vi "PentaPanesDemo.vi"() -> ()   [LabVIEW 2022 SP3]
uses:
  PentaPanesClassLibrary.lvlibp/PanesColors.ctl
  <vilib>/Utility/miscctls.llb/LVBoundsTypeDef.ctl
  Tools/Type Defs/XYZ Indicators.ctl
  Tools/Type Defs/XYZ Controls.ctl
  Tools/Type Defs/XYZ ControlButtonsMini.ctl
  PentaPanesClassLibrary.lvlibp/ResizeBehaviourCluster.ctl
  PentaPanesClassLibrary.lvlibp/BordersCluster.ctl
  PentaPanesClassLibrary.lvlibp/PanePosition.ctl
  <vilib>/Platform/browser.llb/Open URL in Default Browser (string).vi
  PentaPanesClassLibrary.lvlibp/PentaPanes.lvclass
  PentaPanesClassLibrary.lvlibp/1abvi3w/vi.lib/Utility/miscctls.llb/LVBoundsTypeDef.ctl
  PentaPanesClassLibrary.lvlibp
panel:
  out "Logo":picture[](array[picture])
  out "Icons Values":bool[](array[boolean])
  out "IconNames":string[](array[string])
  out "Icons":picture[](array[picture])=[bytes[7230], bytes[7230], bytes[7230], bytes[7230], bytes[7230], bytes[7230], bytes[7230], bytes[7230], bytes[7230], bytes[7230], bytes[7230], bytes[7230], bytes[7230], bytes[7230], bytes[7230], bytes[7230], bytes[7230], bytes[7230], bytes[7230], bytes[7230], bytes[7230], bytes[7230], bytes[7230], bytes[7230], bytes[7230], bytes[7230], bytes[7230], bytes[7230], bytes[7230], bytes[7230], bytes[7230], bytes[7230], bytes[7230], bytes[7230], bytes[7230], bytes[7230], bytes[7230], bytes[7230], bytes[7230], bytes[7230], bytes[7230], bytes[7230], bytes[7230], bytes[7230], bytes[7230], bytes[7230], bytes[7230], bytes[7230], bytes[7230], bytes[7230], bytes[7230], bytes[7230]]
  in  "Options Tree":string[](tree)=["About"]
  in  "Options Tab":T1(tab)
  in  "Developed By\nLEAP CODE\nLinking hardware \nwith software\n\nYoni Cohen":string="yoncoh@gmail.com"
  in  "Icon set by":string="https://icons8.com"
  out "about picture":picture
  in  "Graphs Layout":T2(ring)=enum."3 Line graphs"
  in  "Right Pane View":u16(ring) items=["Simple GUI SubVI", "Positioner", "Debug"]
  in  "Top Pane Size":i32=75 caption="Top"
  in  "Right Pane Size":i32=156 caption="Right" max=4000
  in  "Left Pane Size":i32=113 caption="Left"
  in  "Bottom Pane Size":i32=100 caption="Bottom"
  in  "Colors":T3
  out "Intensity Graph 2":dbl[][](graph)
  out "XY Graph 3":cluster{dbl[], dbl[]}[](graph)
  out "XY Graph 2":cluster{dbl[], dbl[]}[](graph)
  out "XY Graph":cluster{dbl[], dbl[]}[](graph)
  out "Intensity Graph":dbl[][](graph)
  in  "Debug Tab":enum32{"Page 1", "Page 2"}(tab)
  out "Init Error":errorcluster
  out "Eventloop Error":errorcluster
  out "App Path":path=path "E:/Work/5PanesWindow/5PanesDemo.vi"
  out "FP Bounds":T4
  in  "Positioner":enum32{"Page 1", "Page 2"}(tab)
  in  "Directions Cluster 2":T5
  in  "GO Button":bool
  in  "POS 2":T6
  out "POS":T7
  in  "Listbox":i32(listbox)=-1
  # "Overview: A mockup of a GUI window demonstrating the use of \nthe \"PentaPanes\" Class\nRequirements: LabVIEW 2023 or \ncompatible \nInstructions: Run this VI and play \naround with the GUI. \nopen and close panes by pressing the white splitters."
  # "Panes"
  # "Sizes"
  # "Debug Pane"
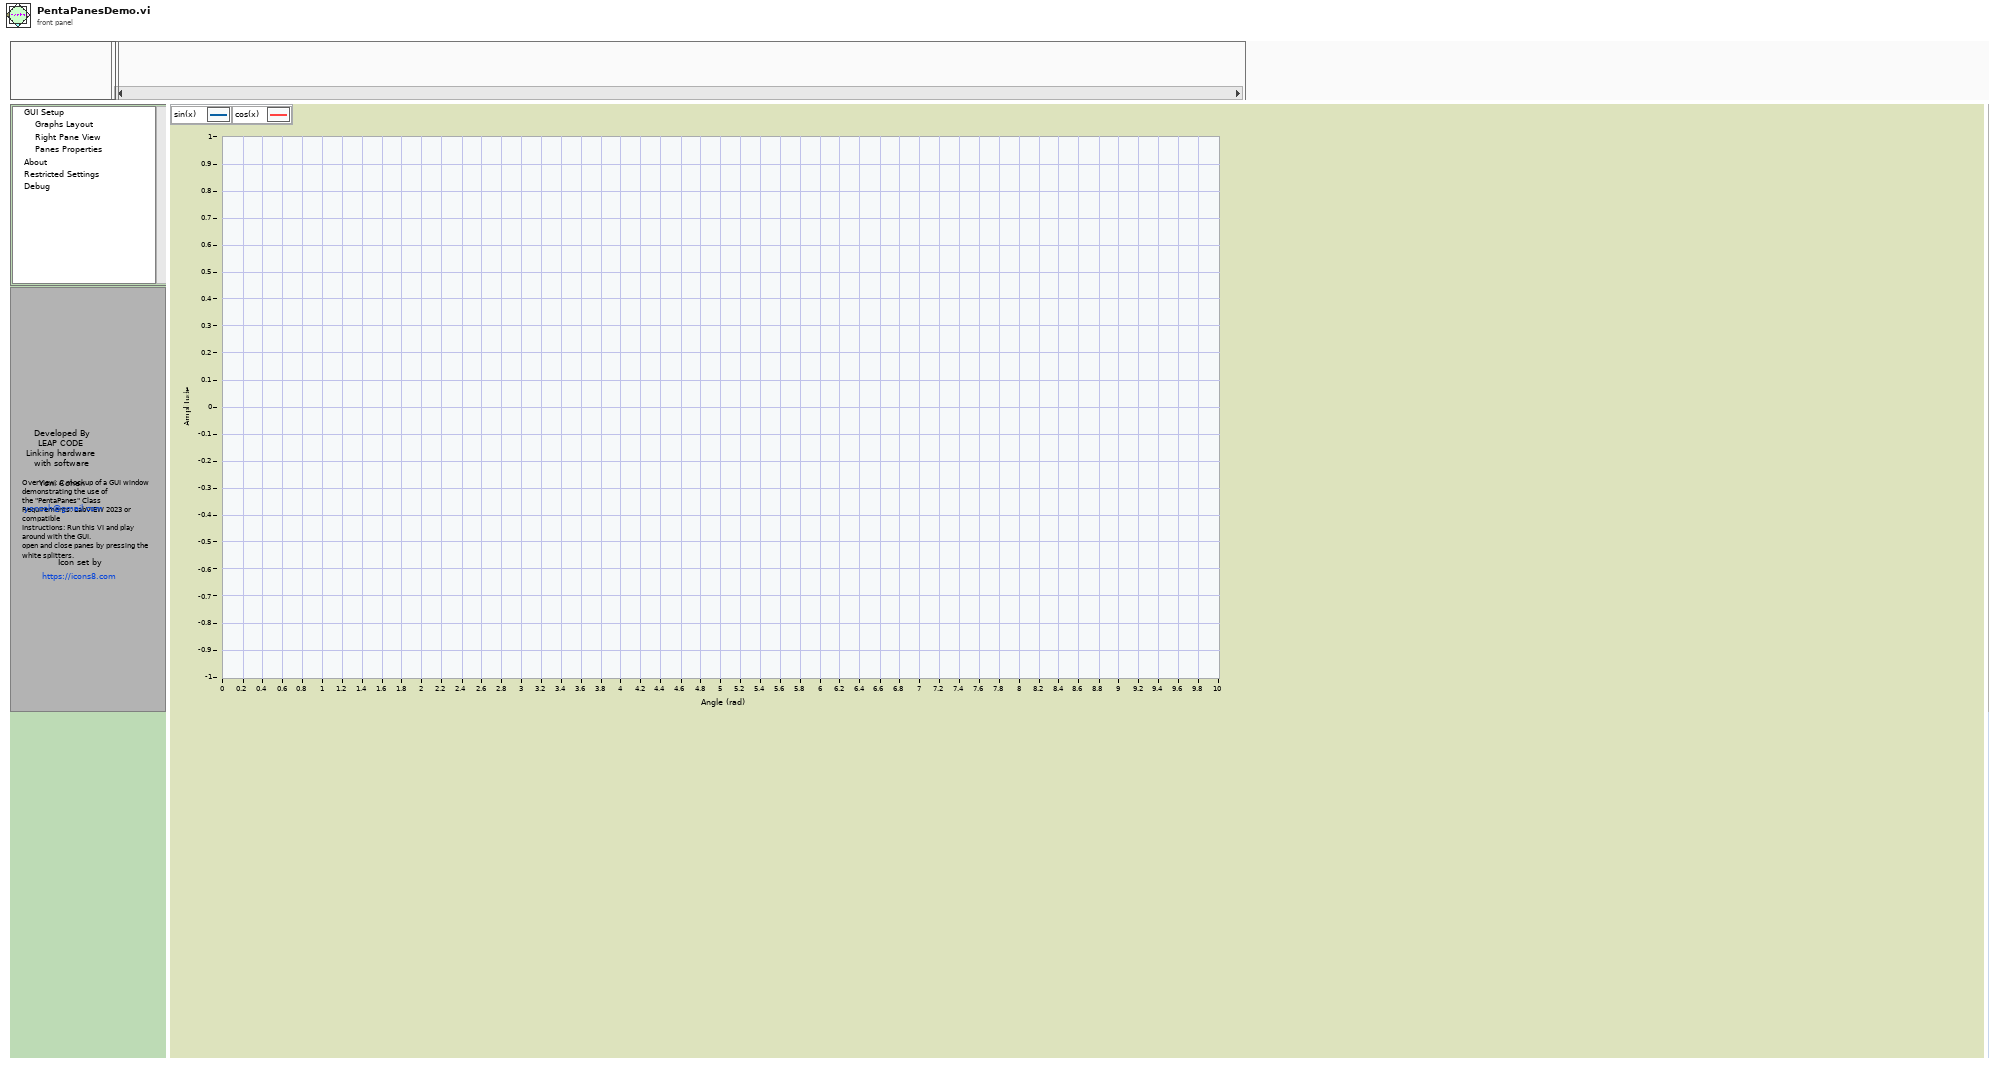
[diagram p1: front panel]
types:
  T1 = enum32{"About", "Graphs Layout", "Right Pane View", "Panes Colors", "Panes Properties", "Debug", "Restricted Settings"}
  T2 = enum16{"1 Line Graph", "1 Line + 2 Intensity", "3 Line graphs", "1 Intensity", "2 Intensity H", "2 Intensity V", "All"}
  T3 = typedef "PentaPanesClassLibrary.lvlibp/PentaPanes.lvclass/PanesColors.ctl" = cluster{"Top Color":u32, "Left Color":u32, "Center Color":u32, "Right Color":u32, "Bottom Color":u32}
  T4 = typedef "LVBoundsTypeDef.ctl" = cluster{"Width":i32, "Height":i32}
  T5 = typedef "XYZ ControlButtonsMini.ctl" = cluster{"Down Button":bool, "Up Button":bool, "Right Button":bool, "Left Button":bool, "In Button":bool, "Out Button":bool}
  T6 = typedef "XYZ Controls.ctl" = cluster{"X":dbl, "Y":dbl, "Z":dbl}
  T7 = typedef "XYZ Indicators.ctl" = cluster{"X":dbl, "Y":dbl, "Z":dbl}
  T8 = enum32{"Invalid", "Standard", "Closed", "Hidden", "Minimized", "Maximized"}
  T9 = enum16{"1 Line Graph", "1 Line + 2 Intensity", "3 Line graphs", "1 Intensity"}
  T10 = enum16{"Always On", "Always Off", "Off While Running"}
  T11 = typedef "PentaPanesClassLibrary.lvlibp/PentaPanes.lvclass/ResizeBehaviourCluster.ctl" = cluster{"Adjust":u16, "Borders":T12, "Borders in Percent?":bool, "Minimal":T13, "Invisible?":bool, "Force aspect ratio?":bool}
  T12 = typedef "PentaPanesClassLibrary.lvlibp/PentaPanes.lvclass/BordersCluster.ctl" = cluster{"Left":i32, "Top":i32, "Right":i32, "Bottom":i32}
  T13 = typedef "PentaPanesClassLibrary.lvlibp/LVBoundsTypeDef.ctl" = cluster{"Width":i32, "Height":i32}
  T14 = cluster{"Adjust":u16, "Borders":T12, "Borders in Percent?":bool, "Minimal":T4, "Invisible?":bool, "Force aspect ratio?":bool}
  T15 = typedef "PentaPanesClassLibrary.lvlibp/PentaPanes.lvclass/PanesCluster.ctl" = cluster{"Top Pane":refnum<vi>, "Left Pane":refnum<vi>, "Center Pane":refnum<vi>, "Right Pane":refnum<vi>, "Bottom Pane":refnum<vi>}
  T16 = cluster{"Left":i32, "Top":i32, "Right":i32, "Bottom":i32}
  T17 = cluster{"Adjust":u16, "Borders":cluster{"Left":i32, "Top":i32, "Right":i32, "Bottom":i32}, "Borders in Percent?":bool, "Minimal":cluster{"Width":u32, "Height":u32}, "Invisible?":bool, "Force aspect ratio?":bool}
  T18 = typedef "LVRectTypeDef.ctl" = cluster{"Left":i16, "Top":i16, "Right":i16, "Bottom":i16}
  T19 = typedef "PentaPanesClassLibrary.lvlibp/PentaPanes.lvclass/PanePosition.ctl" = u16
  T20 = typedef "LVBoundsTypeDef.ctl" = cluster{"Width":u32, "Height":u32}
  T21 = typedef "LVPoint32TypeDef.ctl" = cluster{"Horizontal":i32, "Vertical":i32}
  T22 = typedef "LVRangeTypeDef.ctl" = cluster{"Minimum":dbl, "Maximum":dbl, "Increment":dbl, "Minor Increment":dbl, "Start":dbl}
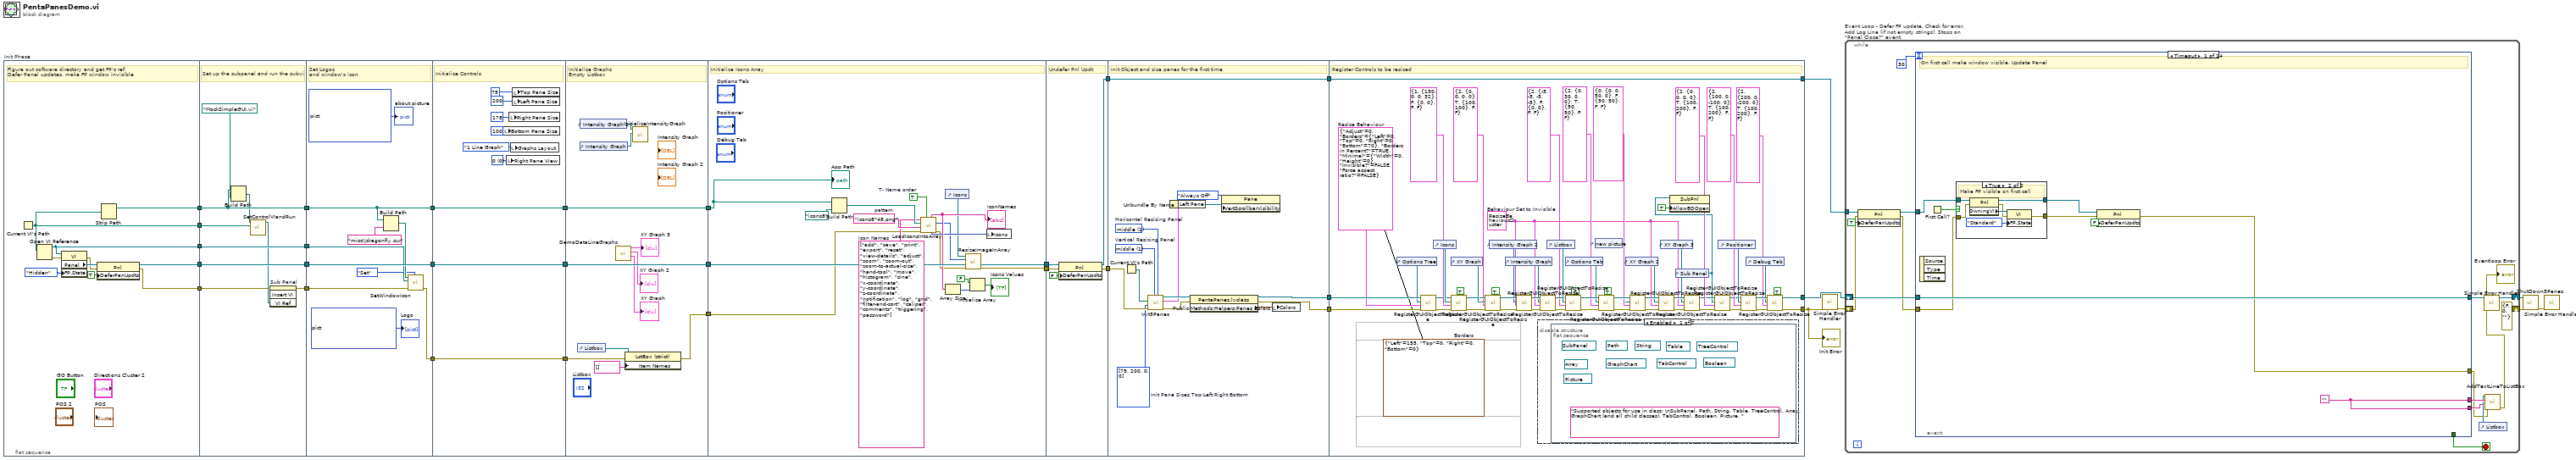
[diagram p0: block diagram]
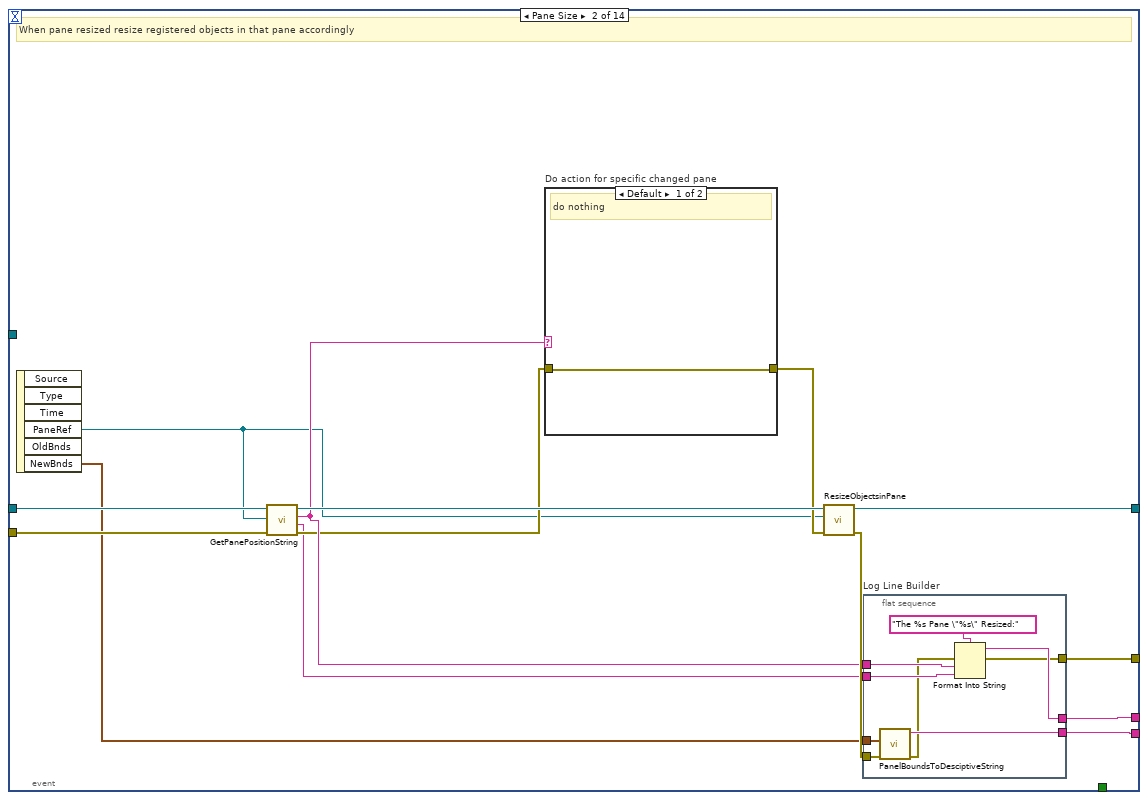
[diagram p4: hidden frame]
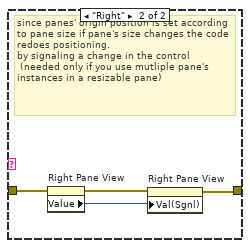
[diagram p5: hidden frame]
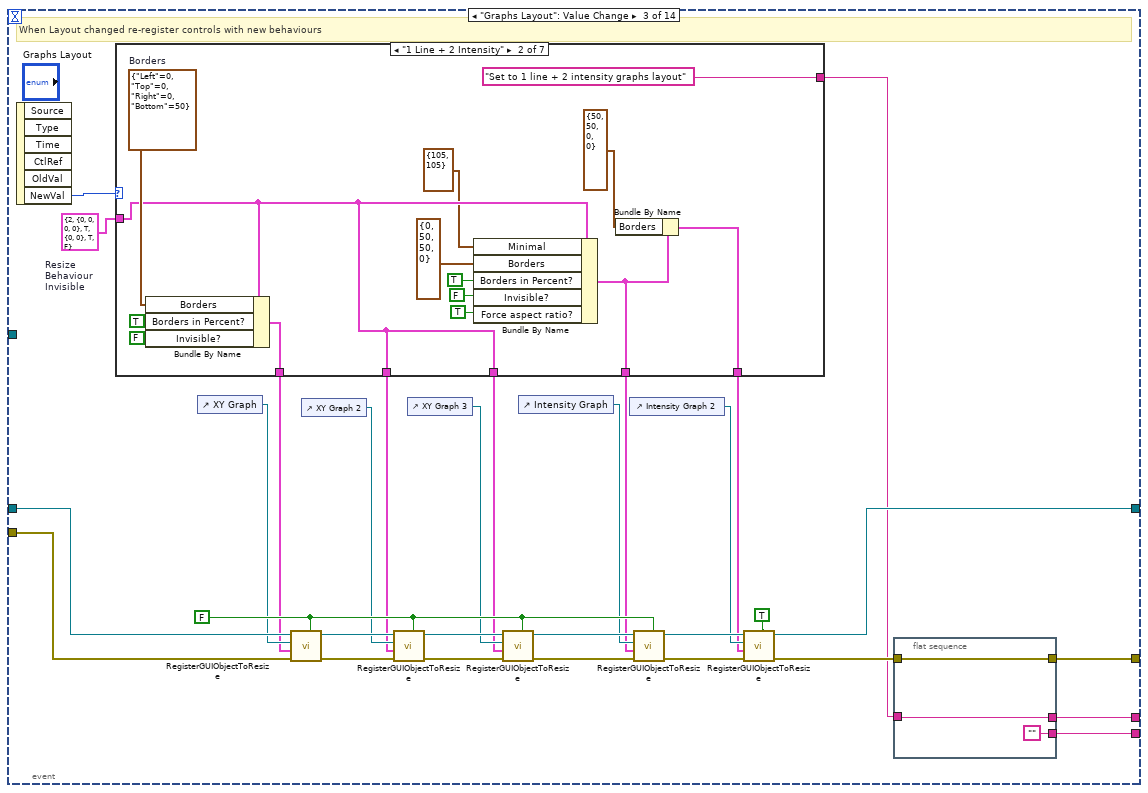
[diagram p6: hidden frame]
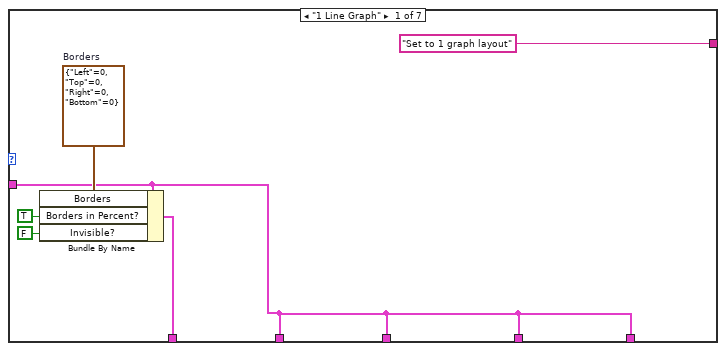
[diagram p7: hidden frame]
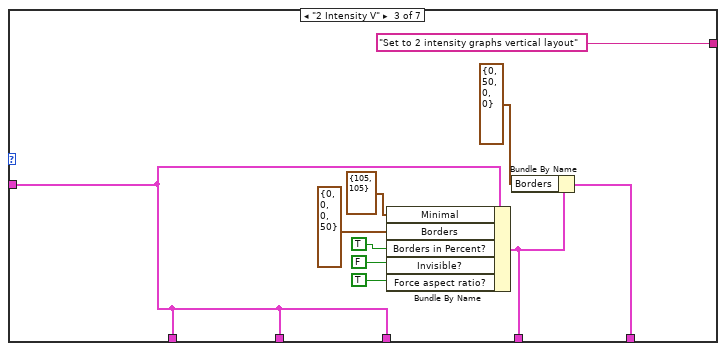
[diagram p8: hidden frame]
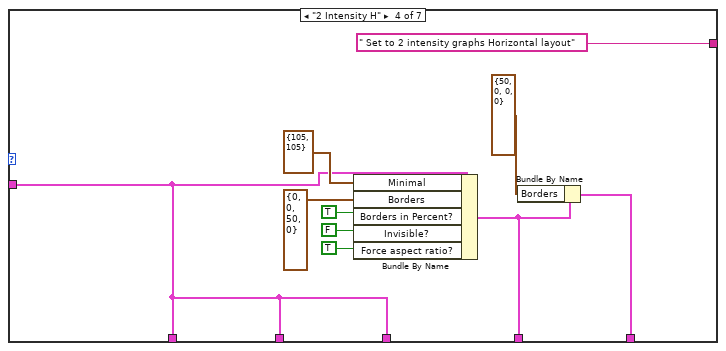
[diagram p9: hidden frame]
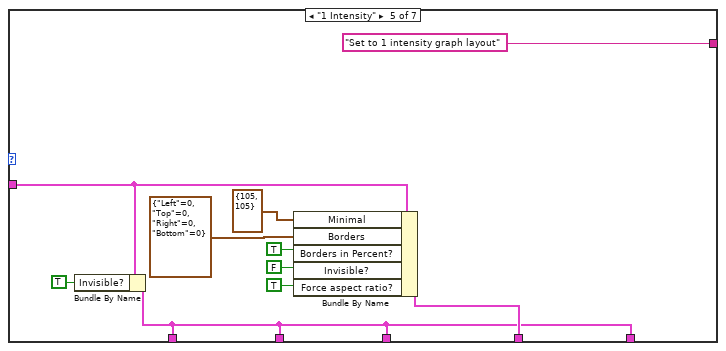
[diagram p10: hidden frame]
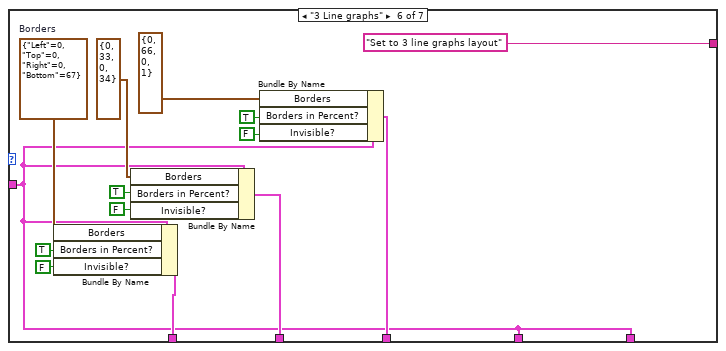
[diagram p11: hidden frame]
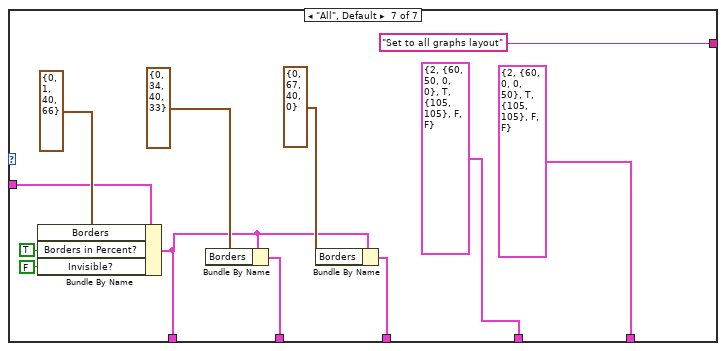
[diagram p12: hidden frame]
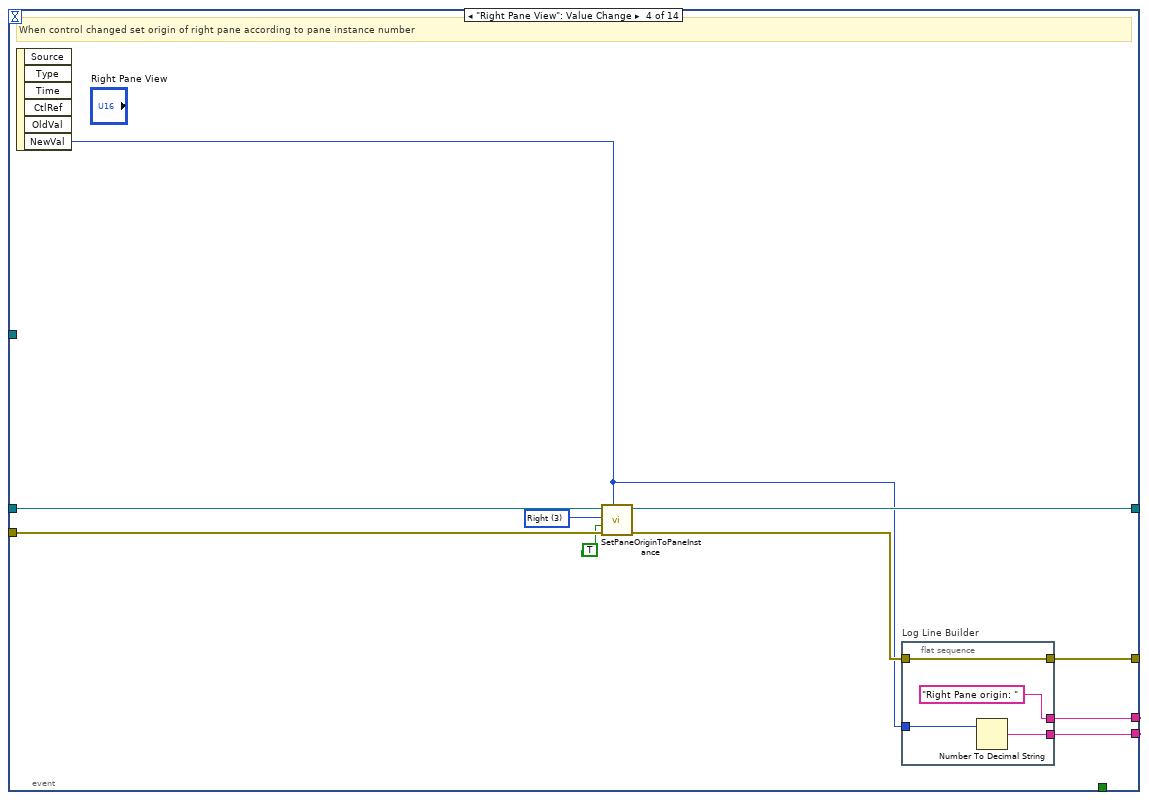
[diagram p13: hidden frame]
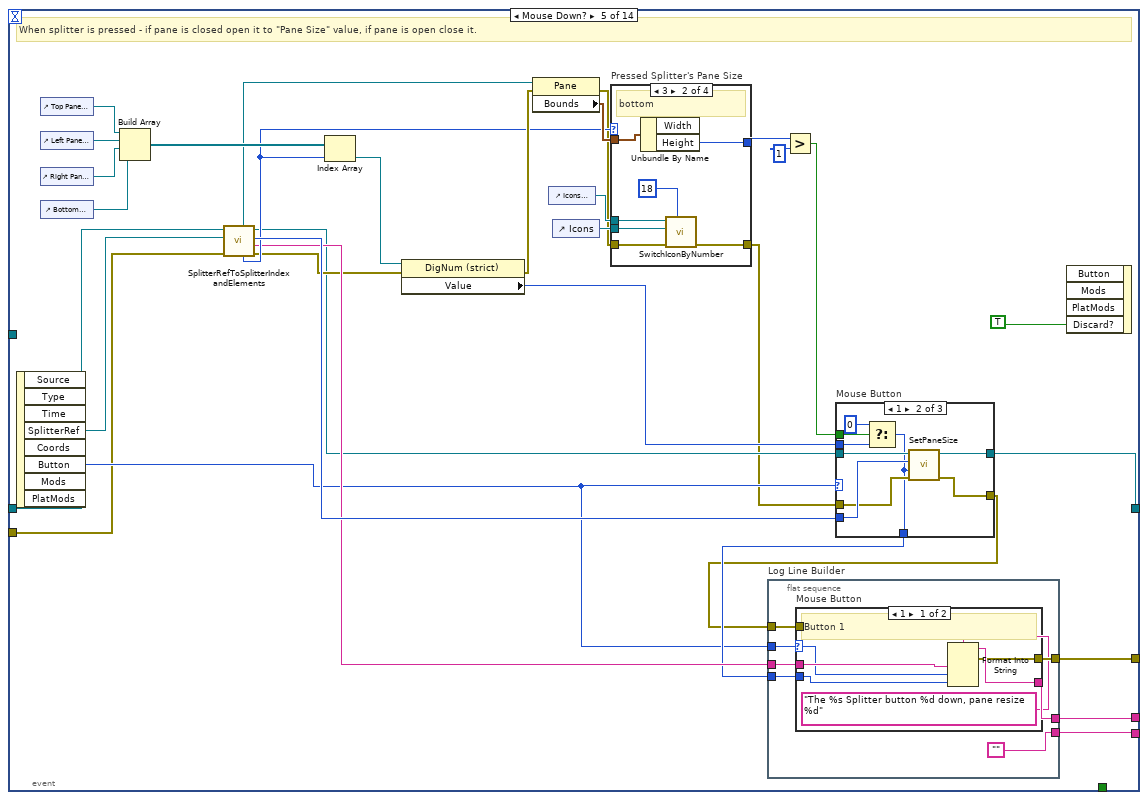
[diagram p14: hidden frame]
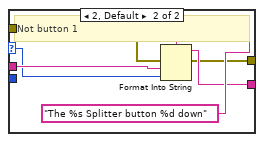
[diagram p15: hidden frame]
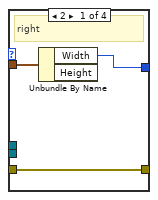
[diagram p16: hidden frame]
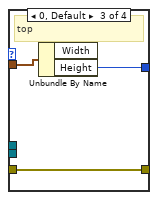
[diagram p17: hidden frame]
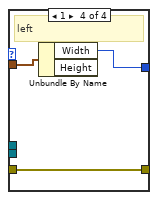
[diagram p18: hidden frame]
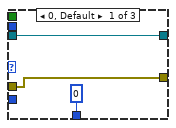
[diagram p19: hidden frame]
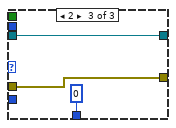
[diagram p20: hidden frame]
diagram:
  n1 = flat-sequence "Init Phase" {
    tunnel: [w39] -> w9
    tunnel: [w37] -> w7
    tunnel: [w36] -> w5
    tunnel: [w34] -> w3
    tunnel: [w33] -> w1
    tunnel: w9 -> [w51]
    tunnel: [w51] -> w8
    tunnel: w7 -> [w47]
    tunnel: [w46] -> w6
    tunnel: w5 -> [w50]
    tunnel: [w50] -> w4
    tunnel: w3 -> [w45]
    tunnel: [w45] -> w2
    tunnel: w1 -> [w49]
    tunnel: [w53] -> w18
    tunnel: w8 -> [w61]
    tunnel: [w61] -> w17
    tunnel: [w58] -> w16
    tunnel: w6 -> [w60]
    tunnel: w4 -> [w59]
    tunnel: w2 -> [w53]
    tunnel: w18 -> [w70]
    tunnel: [w70] -> w24
    tunnel: w17 -> [w69]
    tunnel: [w69] -> w22
    tunnel: [w62] -> w20
    tunnel: w16 -> [w62]
    tunnel: w24 -> [w81]
    tunnel: [w81] -> w23
    tunnel: w22 -> [w80]
    tunnel: [w80] -> w21
    tunnel: w20 -> [w73]
    tunnel: [w72] -> w19
    tunnel: [w98] -> w29
    tunnel: w23 -> [w88]
    tunnel: w21 -> [w98]
    tunnel: [w85] -> w26
    tunnel: w19 -> [w87]
    tunnel: w29 -> [w103]
    tunnel: w26 -> [w101]
    tunnel: [w100] -> w25
    tunnel: [w99] -> w11
    tunnel: [w108] -> w32
    tunnel: [w109] -> w31
    tunnel: w25 -> [w114]
    tunnel: [w107] -> w12
    tunnel: w11 -> [w107]
    tunnel: w32 -> [w141]
    tunnel: w31 -> [w145]
    tunnel: [w136] -> w14
    tunnel: [w135] -> w15
    tunnel: [w121] -> w10
    tunnel: w12 -> [w121]
    frame #0 {
      # "Figure out software directory and get FP's ref,\nDefer Panel updates, make FP window invisible"
      n2 = Current VI's Path() -> (path=w33:path)
      n3 = Open VI Reference(vi path=w33) -> (vi reference=w36:refnum<vi>, error out=w41:errorcluster)  [unwired: 5 in]
      n4 = property on="Property Node" class="VI"(reference=w36, error in=w41, "FP.State"=T8."Hidden" ("Front Panel Window:State")) -> (error out=w38:errorcluster, "Panel"=w42:refnum<vi>)  [unwired: 1 out]
      n5 = property on="Property Node" class="Pnl"(reference=w42, error in=w38, "DeferPanUpdts"=TRUE ("Defer Panel Updates")) -> (reference out=w39:refnum<vi>, error out=w37:errorcluster)
      n6 = Strip Path(path=w33) -> (stripped path=w34:path)  [unwired: 1 out]
    }
    frame #1 {
      # "Set up the subpanel and run the subvi"
      n7 = Build Path(base path=w45, name or relative path=path "MockSimpleGUI.vi" ("stripped path")) -> (appended path=w44:path)
      n8 = call "SetControlVIandRun.vi"("Controlling VI path"=w49, "appended path"=w44) -> ("Sub VI out"=w48:refnum<vi>)  [unwired: 9 in]
      n9 = invoke on="Sub Panel" class="SubPnl" method="Insert VI"(error in=w47, "VI Ref"=w48) -> (error out=w46:errorcluster)  [unwired: 2 in, 3 out]
    }
    frame #2 {
      # "Set Logos \nand window's icon"
      n10 = Build Path(base path=w53, name or relative path="misc\\dragonfly.cur") -> (appended path=w57:path)
      n11 = call "SetWindowIcon.vi"("Action"=enum16{"Set", "Reset"}."Set", "error in (no error)"=w60, "VIRef (calling VI)"=w59, "ICO Icon"=w57) -> ("Error Out"=w58:errorcluster)  [unwired: 7 in]
      "Logo" <- picture[] [bytes[29955]] ("Logo")
      "about picture" <- picture bytes[70768] ("new picture")
    }
    frame #3 {
      w65 = u16 0 items=["0", "1", "2"] ("Right Pane Origin")
      # "Initialize Controls"
      n12 = local write "Bottom Pane Size"(100 ("Bottom Pane Size")) -> ()
      n13 = local write "Right Pane View"(w65) -> ()
      n14 = local write "Right Pane Size"(178 ("Right Pane Size")) -> ()
      n15 = local write "Graphs Layout"(T9."1 Line Graph" ("Graphs Layout")) -> ()
      n16 = local write "Top Pane Size"(75 ("Top Pane Size")) -> ()
      n17 = local write "Left Pane Size"(200 ("Top Pane Size")) -> ()
    }
    frame #4 {
      # "Initialize Graphs\nEmpty Listbox"
      n18 = control-ref of="Listbox"() -> (w71:refnum<vi>)
      n19 = control-ref of="Intensity Graph 2"() -> (w78:refnum<vi>)
      n20 = control-ref of="Intensity Graph"() -> (w79:refnum<vi>)
      n21 = call "DemoDataLineGraphs.vi"() -> (1:"XY Graph 3"=→"XY Graph":cluster{"X":dbl[], "Y":dbl[]}[], "XY Graph 2"=→"XY Graph 2":cluster{"X":dbl[], "Y":dbl[]}[], 3:"XY Graph 3"=→"XY Graph 3":cluster{"X":dbl[], "Y":dbl[]}[])  [unwired: 9 in]
      n22 = property on="Property Node" class="LstBox (strict)"(reference=w71, error in=w73, "Item Names"=string[] []) -> (error out=w72:errorcluster)  [unwired: 1 out]
      n23 = call "InitializeIntensityGraph.vi"("Intensity Graph 1 in"=w79, "IntensityGraph 2 in"=w78) -> ()  [unwired: 10 in]
    }
    frame #5 {
      w83 = TRUE  # T- Name order
      w90 = string[] ["add", "save", "print", "export", "reset", "view-details", "adjust", "zoom", "zoom-out", "zoom-to-actual-size", "hand-tool", "move", "histogram", "sine", "x-coordinate", "y-coordinate", "z-coordinate", "notification", "log", "grid", "filter-and-sort", "caliper", "comments", "triggering", "password"]  # Icon Names
      w91 = "icons8*48.png"  # pattern
      # "Initialize Icons Array"
      n24 = Build Path(base path=w88, name or relative path=path "icons8") -> (appended path=w92:path)
      n25 = call "LoadIconsIntoArray.vi"("T- Name order/F-File order"=w83, "error in"=w87, "Pattern"=w91, "Path to PNG files"=w92, "Name Order in"=w90) -> ("error out"=w86:errorcluster, "Icon Sizes"=w84:i32[], "Icons out"=w89:picture[], "Names out"=w97:string[])  [unwired: 2 in, 1 out]
      "IconNames" <- w97
      n26 = Array Size(array=w97) -> (size(s)=w95:i32)
      n27 = control-ref of="Icons"() -> (w82:refnum<vi>)
      n28 = call "ResizeImageInArray.vi"("error in (no error)"=w86, "Draw Area Width/Height"=w84, "Array in"=w82) -> ("error out"=w85:errorcluster)  [unwired: 8 in]
      n29 = Initialize Array(FALSE, w95) -> (→"Icons Values":bool[])
      n30 = local write "Icons"(w89) -> ()
      "App Path" <- w88
    }
    frame #6 {
      # "Undefer Pnl Updt"
      n31 = property on="Property Node" class="Pnl"(reference=w103, error in=w101, "DeferPanUpdts"=FALSE ("Defer Panel Updates")) -> (reference out=w99:refnum<vi>, error out=w100:errorcluster)
    }
    frame #7 {
      w110 = i32[] [75, 200, 0, 0]  # Init Pane Sizes Top;Left;Right;Bottom
      w115 = u16 1 items=["left", "middle", "right"]  # Horizontal Resizing Panel
      w116 = u16 1 items=["top", "middle", "bottom"]  # Vertical Resizing Panel
      # "Init Object and size panes for the first time"
      n32 = Current VI's Path() -> (path=w113:path)
      n33 = call "Init5Panes.vi"("Horizontal Resizing Pane"=w115, "Vertical Resizing Pane"=w116, "error in (no error)"=w114, "Pane Sizes Top;Left;Right;Bottom"=w110, "Path"=w113) -> ("error out"=w117:errorcluster, "Panes"=w106:T15, "PentaPanesGUI out"=w112:refnum<class "PentaPanes.lvclass">)  [unwired: 4 in]
      n34 = Unbundle By Name(w106) -> ("Left Pane"=w105:refnum<vi>)
      n35 = property on="Property Node" class="PentaPanes.lvclass"(reference=w112, error in=w117) -> (reference out=w109:refnum<class "PentaPanes.lvclass">, error out=w108:errorcluster, "Public Methods:Helpers:Panes Colors"=w111:T3)
      n36 = property class="Pane"(reference=w105, "VertScrollbarVisibility"=T10."Always Off" ("Vertical Scrollbar Visibility")) -> ()  [unwired: 1 in, 2 out]
      n37 = local write "Colors"(w111) -> ()
    }
    frame #8 {
      (unwired) T12 {"Left"=155, "Top"=0, "Right"=0, "Bottom"=0}  # Borders
      w150 = T11 {"Adjust"=2, "Borders"={"Left"=4000, "Top"=0, "Right"=0, "Bottom"=0}, "Borders in Percent?"=FALSE, "Minimal"={"Width"=0, "Height"=0}, "Invisible?"=TRUE, "Force aspect ratio?"=TRUE}  # Behaviour Set to Invisible
      w142 = T11 {"Adjust"=0, "Borders"={"Left"=0, "Top"=0, "Right"=0, "Bottom"=70}, "Borders in Percent?"=TRUE, "Minimal"={"Width"=0, "Height"=0}, "Invisible?"=FALSE, "Force aspect ratio?"=FALSE}  # Resize Behaviour
      # "Register Controls to be resized"
      n38 = control-ref of="Options Tree"() -> (w139:refnum<vi>)
      n39 = call-dynamic "RegisterGUIObjectToResize.vi"("error in (no error)"=w141, "Behaviour"=w142, "Any Control reference"=w139, "PentaPanesGUI in"=w145) -> ("error out"=w127:errorcluster, "PentaPanesGUI out"=w128:refnum<class "PentaPanes.lvclass">)  [unwired: 4 in, 2 out]
      n40 = control-ref of="Icons"() -> (w144:refnum<vi>)
      n41 = control-ref of="XY Graph"() -> (w173:refnum<vi>)
      n42 = call-dynamic "RegisterGUIObjectToResize.vi"("Resize Object?"=TRUE, "error in (no error)"=w127, "Behaviour"=T11 {"Adjust"=1, "Borders"={"Left"=130, "Top"=0, "Right"=0, "Bottom"=32}, "Borders in Percent?"=FALSE, "Minimal"={"Width"=0, "Height"=0}, "Invisible?"=FALSE, "Force aspect ratio?"=FALSE}, "Any Control reference"=w144, "PentaPanesGUI in"=w128) -> ("error out"=w162:errorcluster, "PentaPanesGUI out"=w161:refnum<class "PentaPanes.lvclass">)  [unwired: 3 in, 2 out]
      n43 = call-dynamic "RegisterGUIObjectToResize.vi"("Resize Object?"=TRUE, "error in (no error)"=w162, "Behaviour"=T14 {"Adjust"=2, "Borders"={"Left"=0, "Top"=0, "Right"=0, "Bottom"=0}, "Borders in Percent?"=TRUE, "Minimal"={"Width"=100, "Height"=100}, "Invisible?"=FALSE, "Force aspect ratio?"=FALSE} ("output cluster 2"), "Any Control reference"=w173, "PentaPanesGUI in"=w161) -> ("error out"=w164:errorcluster, "PentaPanesGUI out"=w169:refnum<class "PentaPanes.lvclass">)  [unwired: 3 in, 2 out]
      n44 = control-ref of="Intensity Graph 2"() -> (w149:refnum<vi>)
      n45 = control-ref of="Intensity Graph"() -> (w166:refnum<vi>)
      n46 = call-dynamic "RegisterGUIObjectToResize.vi"("error in (no error)"=w164, "Behaviour"=w150, "Any Control reference"=w149, "PentaPanesGUI in"=w169) -> ("error out"=w165:errorcluster, "PentaPanesGUI out"=w168:refnum<class "PentaPanes.lvclass">)  [unwired: 4 in, 2 out]
      n47 = disable-structure "Diagram Disable Structure" shown="Enabled" {
        frame Enabled {
          n48 = flat-sequence {
            frame #0 {
              (unwired) "Supported objects for use in class: \nSubPanel, Path, String, Table, TreeControl, Array, GraphChart (and all child classes), TabControl, Boolean, Picture. "
              (unwired) refnum<vi> refnum ("XY Graph")
              (unwired) refnum<vi> refnum ("XY Graph")
              (unwired) refnum<vi> refnum ("XY Graph")
              (unwired) refnum<vi> refnum ("XY Graph")
              (unwired) refnum<vi> refnum ("XY Graph")
              (unwired) refnum<vi> refnum ("XY Graph")
              (unwired) refnum<vi> refnum ("XY Graph")
              (unwired) refnum<vi> refnum ("XY Graph")
              (unwired) refnum<vi> refnum ("XY Graph")
              (unwired) refnum<vi> refnum ("XY Graph")
            }
          }
        }
        frame Disabled {
        }
      }
      n49 = call-dynamic "RegisterGUIObjectToResize.vi"("error in (no error)"=w165, "Behaviour"=w150, "Any Control reference"=w166, "PentaPanesGUI in"=w168) -> ("error out"=w163:errorcluster, "PentaPanesGUI out"=w167:refnum<class "PentaPanes.lvclass">)  [unwired: 4 in, 2 out]
      n50 = control-ref of="Listbox"() -> (w172:refnum<vi>)
      n51 = control-ref of="Options Tab"() -> (w140:refnum<vi>)
      n52 = call-dynamic "RegisterGUIObjectToResize.vi"("Resize Object?"=TRUE, "error in (no error)"=w163, "Behaviour"=T11 {"Adjust"=2, "Borders"={"Left"=-5, "Top"=-5, "Right"=-5, "Bottom"=-5}, "Borders in Percent?"=FALSE, "Minimal"={"Width"=0, "Height"=0}, "Invisible?"=FALSE, "Force aspect ratio?"=FALSE} ("output cluster 5"), "Any Control reference"=w172, "PentaPanesGUI in"=w167) -> ("error out"=w174:errorcluster, "PentaPanesGUI out"=w175:refnum<class "PentaPanes.lvclass">)  [unwired: 3 in, 2 out]
      n53 = control-ref of="new picture"() -> (w122:refnum<vi>)
      n54 = call-dynamic "RegisterGUIObjectToResize.vi"("Resize Object?"=TRUE, "error in (no error)"=w174, "Behaviour"=T11 {"Adjust"=2, "Borders"={"Left"=0, "Top"=30, "Right"=0, "Bottom"=0}, "Borders in Percent?"=TRUE, "Minimal"={"Width"=50, "Height"=50}, "Invisible?"=FALSE, "Force aspect ratio?"=FALSE} ("output cluster 6"), "Any Control reference"=w140, "PentaPanesGUI in"=w175) -> ("error out"=w170:errorcluster, "PentaPanesGUI out"=w171:refnum<class "PentaPanes.lvclass">)  [unwired: 3 in, 2 out]
      n55 = control-ref of="XY Graph 2"() -> (w152:refnum<vi>)
      n56 = call-dynamic "RegisterGUIObjectToResize.vi"("error in (no error)"=w170, "Behaviour"=T11 {"Adjust"=0, "Borders"={"Left"=0, "Top"=0, "Right"=50, "Bottom"=0}, "Borders in Percent?"=FALSE, "Minimal"={"Width"=50, "Height"=50}, "Invisible?"=FALSE, "Force aspect ratio?"=FALSE} ("output cluster 7"), "Any Control reference"=w122, "PentaPanesGUI in"=w171) -> ("error out"=w153:errorcluster, "PentaPanesGUI out"=w156:refnum<class "PentaPanes.lvclass">)  [unwired: 4 in, 2 out]
      n57 = call-dynamic "RegisterGUIObjectToResize.vi"("error in (no error)"=w153, "Behaviour"=w150, "Any Control reference"=w152, "PentaPanesGUI in"=w156) -> ("error out"=w154:errorcluster, "PentaPanesGUI out"=w155:refnum<class "PentaPanes.lvclass">)  [unwired: 4 in, 2 out]
      n58 = control-ref of="XY Graph 3"() -> (w151:refnum<vi>)
      n59 = control-ref of="Sub Panel"() -> (w118:refnum<vi>)
      n60 = property class="SubPnl"(reference=w118, "AllowBDOpen"=TRUE ("Allow User to Open Diagram")) -> ()  [unwired: 1 in, 2 out]
      n61 = call-dynamic "RegisterGUIObjectToResize.vi"("error in (no error)"=w154, "Behaviour"=w150, "Any Control reference"=w151, "PentaPanesGUI in"=w155) -> ("error out"=w129:errorcluster, "PentaPanesGUI out"=w132:refnum<class "PentaPanes.lvclass">)  [unwired: 4 in, 2 out]
      n62 = call-dynamic "RegisterGUIObjectToResize.vi"("error in (no error)"=w129, "Behaviour"=T11 {"Adjust"=2, "Borders"={"Left"=0, "Top"=0, "Right"=0, "Bottom"=0}, "Borders in Percent?"=TRUE, "Minimal"={"Width"=100, "Height"=200}, "Invisible?"=FALSE, "Force aspect ratio?"=FALSE}, "Any Control reference"=w118, "PentaPanesGUI in"=w132) -> ("error out"=w130:errorcluster, "PentaPanesGUI out"=w131:refnum<class "PentaPanes.lvclass">)  [unwired: 4 in, 2 out]
      n63 = control-ref of="Positioner"() -> (w148:refnum<vi>)
      n64 = call-dynamic "RegisterGUIObjectToResize.vi"("error in (no error)"=w130, "Behaviour"=T11 {"Adjust"=2, "Borders"={"Left"=100, "Top"=0, "Right"=-100, "Bottom"=0}, "Borders in Percent?"=TRUE, "Minimal"={"Width"=100, "Height"=200}, "Invisible?"=FALSE, "Force aspect ratio?"=FALSE}, "Any Control reference"=w148, "PentaPanesGUI in"=w131) -> ("error out"=w137:errorcluster, "PentaPanesGUI out"=w138:refnum<class "PentaPanes.lvclass">)  [unwired: 4 in, 2 out]
      n65 = control-ref of="Debug Tab"() -> (w134:refnum<vi>)
      n66 = call-dynamic "RegisterGUIObjectToResize.vi"("Resize Object?"=TRUE, "error in (no error)"=w137, "Behaviour"=T11 {"Adjust"=2, "Borders"={"Left"=200, "Top"=0, "Right"=-200, "Bottom"=0}, "Borders in Percent?"=TRUE, "Minimal"={"Width"=100, "Height"=200}, "Invisible?"=FALSE, "Force aspect ratio?"=FALSE}, "Any Control reference"=w134, "PentaPanesGUI in"=w138) -> ("error out"=w136:errorcluster, "PentaPanesGUI out"=w135:refnum<class "PentaPanes.lvclass">)  [unwired: 3 in, 2 out]
    }
  }
  n67 = call <vilib>:"Simple Error Handler.vi"("error in (no error)"=w14) -> ("error out"=w13:errorcluster)  [unwired: 4 in, 4 out]
  n68 = while "Event Loop - Defer FP update, Check for error. Add Log Line (if not empty strings). Stops on \"Panel Close?\" event." {
    shift-right: [w188] -> w28
    shift-left: w15 -> [w189]
    shift-right: [errorcluster {"status"=FALSE, "code"=0, "source"=""} ("error out")] -> w30
    shift-left: w13 -> [w183]
    tunnel: w10 -> [w180]
    stop <- w190 stop-if-true
    n69 = property on="Property Node" class="Pnl"(reference=w180, error in=w183, "DeferPanUpdts"=TRUE ("Defer Panel Updates")) -> (reference out=w182:refnum<vi>, error out=w184:errorcluster)
    n70 = event shown="[0] Timeout" {
      selector: _ -> [_ _ _ _ _ _ _ _ _ _ _ _ _ _]
      dyn-events: _ -> [_ _ _ _ _ _ _ _ _ _ _ _ _ _]
      timeout: 30 -> [_ _ _ _ _ _ _ _ _ _ _ _ _ _]
      tunnel: [_ _ _ _ _ _ _ _ _ TRUE _ _ _ _] -> w190
      tunnel: w189 -> [w199 w220 w263 w355 w369 w447 w483 w502 w624 w638 w652 w677 w688 w701]
      tunnel: w184 -> [w194 w218 w250 w354 w364 w455 w481 w491 w615 w637 w644 w675 w685 w696]
      tunnel: [w199 w221 w253 w350 w392 w456 w482 w503 w624 w638 w651 w676 w688 w701] -> w188
      tunnel: [w196 w215 w264 w351 w370 w457 w476 w504 w625 w637 w653 w671 w687 w699] -> w178
      tunnel: [w198 w214 w265 w352 w377 w458 w478 w509 w626 "" ("String") w654 w673 w684 w697] -> w179
      tunnel: [w198 w222 w266 w353 w376 w459 w479 w508 w627 "VI closed" ("String") w655 w670 w686 "Opening icon set creator website: " ("String")] -> w187
      tunnel: w182 -> [w191 _ _ _ _ _ _ w495 _ _ _ _ _ _]
      event Timeout {
        w198 = "" ("Empty String Constant")
        # "On first call make window visible. Update Panel"
        n71 = event-data() -> ()  [unwired: 1 in, 3 out]
        n72 = First Call?() -> (First Call?: T/F=w195:bool)
        n73 = case shown="True" w195 {
          tunnel: w191 -> [w200 w208]
          tunnel: w194 -> [w201 w205]
          tunnel: [w201 w203] -> w193
          tunnel: [w200 w202] -> w192
          frame False {
          }
          frame True {
            # "Make FP visible on first call"
            n74 = property on="Property Node" class="Pnl"(reference=w208, error in=w205) -> (reference out=w202:refnum<vi>, error out=w204:errorcluster, "OwningVI"=w207:refnum<vi>)
            n75 = property class="VI"(reference=w207, error in=w204, "FP.State"=T8."Standard" ("Front Panel Window:State")) -> (error out=w203:errorcluster)  [unwired: 1 out]
          }
        }
        n76 = property on="Property Node" class="Pnl"(reference=w192, error in=w193, "DeferPanUpdts"=FALSE ("Defer Panel Updates")) -> (error out=w196:errorcluster)  [unwired: 1 out]
      }
      event Pane Size {
        # "When pane resized resize registered objects in that pane accordingly"
        n77 = event-data() -> ("PaneRef"=w209:refnum<vi>, "NewBnds"=w216:T18)  [unwired: 1 in, 4 out]
        n78 = call "GetPanePositionString.vi"("error in (no error)"=w218, "PaneRef"=w209, "PentaPanesGUI in"=w220) -> ("error out"=w212:errorcluster, "Label.Text"=w210:string, "Pos String"=w213:string, "PentaPanesGUI out"=w219:refnum<class "PentaPanes.lvclass">)  [unwired: 5 in]
        n79 = case "Do action for specific changed pane" shown="Default" w213 {
          tunnel: w212 -> [w223 w226]
          tunnel: [w223 w224] -> w211
          frame Default {
            # "do nothing"
          }
          frame "Right" {
            # "since panes' origin position is set according to pane size if pane's size changes the code redoes positioning.\nby signaling a change in the control\n (needed only if you use mutliple pane's instances in a resizable pane)"
            n80 = property on="Right Pane View" class="Ring (strict)"(error in=w226) -> (error out=w225:errorcluster, "Value"=w227:u16)  [unwired: 1 in, 1 out]
            n81 = property on="Right Pane View" class="Ring (strict)"(error in=w225, "Val(Sgnl)"=w227) -> (error out=w224:errorcluster)  [unwired: 1 in, 1 out]
          }
        }
        n82 = call-dynamic "ResizeObjectsinPane.vi"("error in (no error)"=w211, "PaneRef"=w209, "PentaPanesGUI in"=w219) -> ("error out"=w217:errorcluster, "PentaPanesGUI out"=w221:refnum<class "PentaPanes.lvclass">)  [unwired: 7 in]
        n83 = flat-sequence "Log Line Builder" {
          tunnel: [w232] -> w222
          tunnel: w217 -> [w236]
          tunnel: w216 -> [w235]
          tunnel: [w228] -> w215
          tunnel: [w234] -> w214
          tunnel: w213 -> [w231]
          tunnel: w210 -> [w230]
          frame #0 {
            n84 = call "PanelBoundsToDesciptiveString.vi"("error in (no error)"=w236, "Panel Bounds"=w235) -> ("error out"=w229:errorcluster, "String"=w234:string)  [unwired: 8 in]
            n85 = Format Into String(format string="The %s Pane \"%s\" Resized:", error in=w229, w231, w230) -> (resulting string=w232:string, error out=w228:errorcluster)  [unwired: 1 in]
          }
        }
      }
      event "Graphs Layout": Value Change {
        w247 = T11 {"Adjust"=2, "Borders"={"Left"=0, "Top"=0, "Right"=0, "Bottom"=0}, "Borders in Percent?"=TRUE, "Minimal"={"Width"=0, "Height"=0}, "Invisible?"=TRUE, "Force aspect ratio?"=FALSE}  # Resize  Behaviour Invisible
        w256 = FALSE ("Resize Object?")
        # "When Layout changed re-register controls with new behaviours"
        n86 = event-data() -> ("NewVal"=w246:T2)  [unwired: 1 in, 5 out]
        n87 = case shown="\"1 Line + 2 Intensity\"" w246 {
          tunnel: [w267 w275 w288 w298 w312 w317 T17 {"Adjust"=2, "Borders"={"Left"=60, "Top"=50, "Right"=0, "Bottom"=0}, "Borders in Percent?"=TRUE, "Minimal"={"Width"=105, "Height"=105}, "Invisible?"=FALSE, "Force aspect ratio?"=FALSE} ("output cluster")] -> w242
          tunnel: [w269 w283 w287 w297 w308 w327 w331] -> w245
          tunnel: ["Set to 1 graph layout" ("String") "Set to 1 line + 2 intensity graphs layout" ("String") "Set to 2 intensity graphs vertical layout" ("String") " Set to 2 intensity graphs Horizontal layout" ("String") "Set to 1 intensity graph layout" ("String") "Set to 3 line graphs layout" ("String") "Set to all graphs layout" ("String")] -> w248
          tunnel: w247 -> [w267 w274 w287 w297 w310 w317 w335]
          tunnel: [w267 w277 w291 w301 w308 w317 T17 {"Adjust"=2, "Borders"={"Left"=60, "Top"=0, "Right"=0, "Bottom"=50}, "Borders in Percent?"=TRUE, "Minimal"={"Width"=105, "Height"=105}, "Invisible?"=FALSE, "Force aspect ratio?"=FALSE} ("output cluster 2")] -> w241
          tunnel: [w267 w274 w287 w297 w308 w322 w332] -> w237
          tunnel: [w267 w274 w287 w297 w308 w321 w337] -> w238
          frame "1 Line Graph" {
            w268 = T16 {"Left"=0, "Top"=0, "Right"=0, "Bottom"=0}  # Borders
            n88 = Bundle By Name(cluster=w267, "Borders"=w268, "Borders in Percent?"=TRUE, "Invisible?"=FALSE) -> (w269:T11)
          }
          frame "1 Line + 2 Intensity" {
            w285 = T16 {"Left"=0, "Top"=0, "Right"=0, "Bottom"=50}  # Borders
            n89 = Bundle By Name(cluster=w274, "Borders"=w285, "Borders in Percent?"=TRUE, "Invisible?"=FALSE) -> (w283:T11)
            n90 = Bundle By Name(cluster=w274, "Minimal"=T4 {"Width"=105, "Height"=105}, "Borders"=T12 {"Left"=0, "Top"=50, "Right"=50, "Bottom"=0}, "Borders in Percent?"=TRUE, "Invisible?"=FALSE, "Force aspect ratio?"=TRUE ("Force Aspect Ratio?")) -> (w275:T11)
            n91 = Bundle By Name(cluster=w275, "Borders"=T16 {"Left"=50, "Top"=50, "Right"=0, "Bottom"=0}) -> (w277:T11)
          }
          frame "2 Intensity V" {
            n92 = Bundle By Name(cluster=w287, "Minimal"=cluster{"Width":u32, "Height":u32} {"Width"=105, "Height"=105}, "Borders"=T16 {"Left"=0, "Top"=0, "Right"=0, "Bottom"=50}, "Borders in Percent?"=TRUE, "Invisible?"=FALSE, "Force aspect ratio?"=TRUE ("Force Aspect Ratio?")) -> (w288:T11)
            n93 = Bundle By Name(cluster=w288, "Borders"=T16 {"Left"=0, "Top"=50, "Right"=0, "Bottom"=0}) -> (w291:T11)
          }
          frame "2 Intensity H" {
            n94 = Bundle By Name(cluster=w297, "Minimal"=cluster{"Width":u32, "Height":u32} {"Width"=105, "Height"=105}, "Borders"=T16 {"Left"=0, "Top"=0, "Right"=50, "Bottom"=0}, "Borders in Percent?"=TRUE, "Invisible?"=FALSE, "Force aspect ratio?"=TRUE ("Force Aspect Ratio?")) -> (w298:T11)
            n95 = Bundle By Name(cluster=w298, "Borders"=T16 {"Left"=50, "Top"=0, "Right"=0, "Bottom"=0}) -> (w301:T11)
          }
          frame "1 Intensity" {
            n96 = Bundle By Name(cluster=w310, "Invisible?"=TRUE) -> (w308:T11)
            n97 = Bundle By Name(cluster=w310, "Minimal"=cluster{"Width":u32, "Height":u32} {"Width"=105, "Height"=105}, "Borders"=T16 {"Left"=0, "Top"=0, "Right"=0, "Bottom"=0}, "Borders in Percent?"=TRUE, "Invisible?"=FALSE, "Force aspect ratio?"=TRUE ("Force Aspect Ratio?")) -> (w312:T11)
          }
          frame "3 Line graphs" {
            w329 = T16 {"Left"=0, "Top"=0, "Right"=0, "Bottom"=67}  # Borders
            n98 = Bundle By Name(cluster=w317, "Borders"=w329, "Borders in Percent?"=TRUE, "Invisible?"=FALSE) -> (w327:T11)
            n99 = Bundle By Name(cluster=w317, "Borders"=T16 {"Left"=0, "Top"=33, "Right"=0, "Bottom"=34}, "Borders in Percent?"=TRUE, "Invisible?"=FALSE) -> (w322:T11)
            n100 = Bundle By Name(cluster=w317, "Borders"=T16 {"Left"=0, "Top"=66, "Right"=0, "Bottom"=1}, "Borders in Percent?"=TRUE, "Invisible?"=FALSE) -> (w321:T11)
          }
          frame "All", Default {
            n101 = Bundle By Name(cluster=w335, "Borders"=T12 {"Left"=0, "Top"=1, "Right"=40, "Bottom"=66}, "Borders in Percent?"=TRUE, "Invisible?"=FALSE) -> (w331:T11)
            n102 = Bundle By Name(cluster=w331, "Borders"=T16 {"Left"=0, "Top"=34, "Right"=40, "Bottom"=33}) -> (w332:T11)
            n103 = Bundle By Name(cluster=w331, "Borders"=T16 {"Left"=0, "Top"=67, "Right"=40, "Bottom"=0}) -> (w337:T11)
          }
        }
        n104 = control-ref of="XY Graph"() -> (w251:refnum<vi>)
        n105 = call-dynamic "RegisterGUIObjectToResize.vi"("Resize Object?"=w256, "error in (no error)"=w250, "Behaviour"=w245, "Any Control reference"=w251, "PentaPanesGUI in"=w263) -> ("error out"=w262:errorcluster, "PentaPanesGUI out"=w261:refnum<class "PentaPanes.lvclass">)  [unwired: 3 in, 2 out]
        n106 = control-ref of="XY Graph 2"() -> (w239:refnum<vi>)
        n107 = call-dynamic "RegisterGUIObjectToResize.vi"("Resize Object?"=w256, "error in (no error)"=w262, "Behaviour"=w237, "Any Control reference"=w239, "PentaPanesGUI in"=w261) -> ("error out"=w259:errorcluster, "PentaPanesGUI out"=w260:refnum<class "PentaPanes.lvclass">)  [unwired: 3 in, 2 out]
        n108 = control-ref of="XY Graph 3"() -> (w240:refnum<vi>)
        n109 = call-dynamic "RegisterGUIObjectToResize.vi"("Resize Object?"=w256, "error in (no error)"=w259, "Behaviour"=w238, "Any Control reference"=w240, "PentaPanesGUI in"=w260) -> ("error out"=w257:errorcluster, "PentaPanesGUI out"=w258:refnum<class "PentaPanes.lvclass">)  [unwired: 3 in, 2 out]
        n110 = control-ref of="Intensity Graph"() -> (w243:refnum<vi>)
        n111 = control-ref of="Intensity Graph 2"() -> (w244:refnum<vi>)
        n112 = call-dynamic "RegisterGUIObjectToResize.vi"("Resize Object?"=w256, "error in (no error)"=w257, "Behaviour"=w242, "Any Control reference"=w243, "PentaPanesGUI in"=w258) -> ("error out"=w254:errorcluster, "PentaPanesGUI out"=w255:refnum<class "PentaPanes.lvclass">)  [unwired: 3 in, 2 out]
        n113 = call-dynamic "RegisterGUIObjectToResize.vi"("Resize Object?"=TRUE, "error in (no error)"=w254, "Behaviour"=w241, "Any Control reference"=w244, "PentaPanesGUI in"=w255) -> ("error out"=w252:errorcluster, "PentaPanesGUI out"=w253:refnum<class "PentaPanes.lvclass">)  [unwired: 3 in, 2 out]
        n114 = flat-sequence {
          tunnel: [w343] -> w266
          tunnel: ["" ("Empty String Constant")] -> w265
          tunnel: w252 -> [w345]
          tunnel: [w345] -> w264
          tunnel: w248 -> [w343]
          frame #0 {
          }
        }
      }
      event "Right Pane View": Value Change {
        w348 = u16 3 items=["Top", "Left", "Center", "Right", "Bottom"] ("Pane")
        # "When control changed set origin of right pane according to pane instance number"
        n115 = event-data() -> ("NewVal"=w347:u16)  [unwired: 1 in, 5 out]
        n116 = call "SetPaneOriginToPaneInstance.vi"("Pane number"=w347, "error in (no error)"=w354, "Panes Origin differ by - X(T) or Y(F)"=TRUE, "Pane"=w348, "PentaPanesGUI in"=w355) -> ("error out"=w349:errorcluster, "PentaPanesGUI out"=w350:refnum<class "PentaPanes.lvclass">)  [unwired: 5 in]
        n117 = flat-sequence "Log Line Builder" {
          tunnel: w347 -> [w359]
          tunnel: ["Right Pane origin: " ("String")] -> w353
          tunnel: [w357] -> w352
          tunnel: w349 -> [w356]
          tunnel: [w356] -> w351
          frame #0 {
            n118 = Number To Decimal String(number=w359) -> (decimal integer string=w357:string)  [unwired: 1 in]
          }
        }
      }
      event Mouse Down? {
        # "When splitter is pressed - if pane is closed open it to \"Pane Size\" value, if pane is open close it."
        n119 = event-data() -> ("SplitterRef"=w366:refnum<vi>, "Button"=w372:u16)  [unwired: 1 in, 6 out]
        n120 = control-ref of="Top Pane Size"() -> (w391:refnum<vi>)
        n121 = control-ref of="Left Pane Size"() -> (w390:refnum<vi>)
        n122 = control-ref of="Right Pane Size"() -> (w389:refnum<vi>)
        n123 = control-ref of="Bottom Pane Size"() -> (w388:refnum<vi>)
        n124 = Build Array(w391, w390, w389, w388) -> (w387:refnum<vi>[])
        n125 = call "SplitterRefToSplitterIndexandElements.vi"("error in (no error)"=w364, "SplitterRef"=w366, "PentaPanesGUI in"=w369) -> ("error out"=w368:errorcluster, "Splitter String"=w374:string, "Splitter Pane Pos"=w383:T19, "PentaPanesGUI out"=w367:refnum<class "PentaPanes.lvclass">, "Pressed Splitter Index Out"=w375:i32, "Pane Ref out"=w380:refnum<vi>)  [unwired: 3 in]
        n126 = Index Array(array=w387, index=w375) -> (element=w365:refnum<vi>)
        n127 = property on="Property Node" class="DigNum (strict)"(reference=w365, error in=w368) -> (error out=w378:errorcluster, "Value"=w386:i32)  [unwired: 1 out]
        n128 = property on="Property Node" class="Pane"(reference=w380, error in=w378) -> (error out=w361:errorcluster, "Bounds"=w384:T20)  [unwired: 1 out]
        n129 = control-ref of="Icons Values"() -> (w362:refnum<vi>)
        n130 = control-ref of="Icons"() -> (w363:refnum<vi>)
        n131 = case "Pressed Splitter's Pane Size" shown="3" w375 {
          tunnel: w384 -> [w414 w421 w424 w427]
          tunnel: [w413 w420 w423 w426] -> w382
          tunnel: w363 -> [_ w418 _ _]
          tunnel: w362 -> [_ w417 _ _]
          tunnel: w361 -> [w412 w416 w422 w425]
          tunnel: [w412 w415 w422 w425] -> w360
          frame 2 {
            # "right"
            n132 = Unbundle By Name(w414) -> ("Width"=w413:u32)  [unwired: 1 out]
          }
          frame 3 {
            # "bottom"
            n133 = Unbundle By Name(w421) -> ("Height"=w420:u32)  [unwired: 1 out]
            n134 = call "SwitchIconByNumber.vi"("Index"=u32 18, "error in (no error)"=w416, "Icon Array Ref"=w418, "Switch Values ref"=w417) -> ("error out"=w415:errorcluster)  [unwired: 4 in, 3 out]
          }
          frame 0, Default {
            # "top"
            n135 = Unbundle By Name(w424) -> ("Height"=w423:u32)  [unwired: 1 out]
          }
          frame 1 {
            # "left"
            n136 = Unbundle By Name(w427) -> ("Width"=w426:u32)  [unwired: 1 out]
          }
        }
        n137 = flat-sequence "Log Line Builder" {
          tunnel: [w399] -> w376
          tunnel: [w397] -> w370
          tunnel: ["" ("String")] -> w377
          tunnel: w374 -> [w398]
          tunnel: w373 -> [w396]
          tunnel: w372 -> [w394]
          tunnel: w371 -> [w393]
          frame #0 {
            n138 = case "Mouse Button" shown="1" w394 {
              selector: w394 -> [w400 w406]
              tunnel: [w404 w410] -> w399
              tunnel: w398 -> [w403 w409]
              tunnel: [w402 w408] -> w397
              tunnel: w396 -> [w401 _]
              tunnel: w393 -> [_ w407]
              frame 1 {
                # "Button 1"
                n139 = Format Into String(format string="The %s Splitter button %d down, pane resize %d", w403, w400, w401) -> (resulting string=w404:string, error out=w402:errorcluster)  [unwired: 2 in]
              }
              frame 2, Default {
                # "Not button 1"
                n140 = Format Into String(format string="The %s Splitter button %d down", error in=w407, w409, w406) -> (resulting string=w410:string, error out=w408:errorcluster)  [unwired: 1 in]
              }
            }
          }
        }
        n141 = Greater?(x=w382, y=u32 1) -> (0:w379:bool)
        n142 = case "Mouse Button" shown="1" w372 {
          tunnel: w367 -> [w430 w439 w441]
          tunnel: [w430 w438 w441] -> w392
          tunnel: w383 -> [_ w437 _]
          tunnel: w386 -> [_ w432 _]
          tunnel: w360 -> [w429 w435 w442]
          tunnel: [w429 w436 w442] -> w371
          tunnel: w379 -> [_ w434 _]
          tunnel: [0 ("Value") w431 0 ("Value")] -> w373
          frame 0, Default {
          }
          frame 1 {
            n143 = Select(t=i16 0, s=w434, f=w432) -> (s? t:f=w431:i32)
            n144 = call "SetPaneSize.vi"("error in (no error)"=w435, "Pane Size"=w431, "Pane Position"=w437, "PentaPanesGUI in"=w439) -> ("error out"=w436:errorcluster, "PentaPanesGUI out"=w438:refnum<class "PentaPanes.lvclass">)  [unwired: 6 in]
          }
          frame 2 {
          }
        }
        n145 = event-data ("Event Filter Node")("Discard?"=TRUE) -> ()  [unwired: 4 in, 1 out]
      }
      event "Left Pane Size", "Top Pane Size", "Right Pane Size", "Bottom Pane Size": Value Change {
        # "When one of the \"Size\" controls' value changed set appropriate pane size"
        n146 = control-ref of="Top Pane Size"() -> (w454:refnum<vi>)
        n147 = control-ref of="Left Pane Size"() -> (w453:refnum<vi>)
        n148 = control-ref of="Bottom Pane Size"() -> (w450:refnum<vi>)
        n149 = event-data() -> ("CtlRef"=w448:refnum<vi>, "NewVal"=w446:i32)  [unwired: 1 in, 4 out]
        n150 = control-ref of="Right Pane Size"() -> (w451:refnum<vi>)
        n151 = Build Array(w454, w453, refnum<vi> refnum ("element"), w451, w450) -> (w449:refnum<vi>[])
        n152 = Search 1D Array(1D array=w449, element=w448) -> (index of element=w444:i32)  [unwired: 1 in]
        n153 = case shown="True" TRUE {
          tunnel: [w461 w467] -> w456
          tunnel: w455 -> [w460 w466]
          tunnel: w447 -> [w461 w465]
          tunnel: w446 -> [_ w464]
          tunnel: [w460 w462] -> w445
          tunnel: w444 -> [_ w463]
          frame False {
          }
          frame True {
            n154 = call "SetPaneSize.vi"("error in (no error)"=w466, "Pane Size"=w464, "Pane Position"=w463, "PentaPanesGUI in"=w465) -> ("error out"=w462:errorcluster, "PentaPanesGUI out"=w467:refnum<class "PentaPanes.lvclass">)  [unwired: 6 in]
          }
        }
        n155 = flat-sequence "Log Line Builder" {
          tunnel: w446 -> [w468]
          tunnel: [w473] -> w459
          tunnel: [w475] -> w458
          tunnel: [w471] -> w457
          tunnel: w445 -> [w471]
          tunnel: w444 -> [w469]
          frame #0 {
            n156 = Index Array(array=string[] ["Top", "Left", "Center", "Right", "Bottom"], index=w469) -> (element=w472:string)
            n157 = Concatenate Strings(w472, " Pane resized: " ("String")) -> (w473:string)
            n158 = Number To Decimal String(number=w468) -> (decimal integer string=w475:string)  [unwired: 1 in]
          }
        }
      }
      event Value Change {
        # "When Pane Colors Change - Set to new pane colors"
        n159 = event-data() -> ("CtlRef"=w484:refnum<vi>, "NewVal"=w480:T3)  [unwired: 1 in, 4 out]
        n160 = call-dynamic "SetColors.vi"("error in (no error)"=w481, "Colors"=w480, "PentaPanesGUI in"=w483) -> ("error out"=w477:errorcluster, "PentaPanesGUI out"=w482:refnum<class "PentaPanes.lvclass">)  [unwired: 7 in]
        n161 = flat-sequence "Log Line Builder" {
          tunnel: w484 -> [w489]
          tunnel: ["Panes colors set to " ("String")] -> w479
          tunnel: [w487] -> w478
          tunnel: w477 -> [w486]
          tunnel: [w485] -> w476
          frame #0 {
            n162 = call "ClusterToDescriptiveString.vi"("error in"=w486, "Cluster In"=w489) -> ("error out"=w485:errorcluster, "String"=w487:string)  [unwired: 8 in]
          }
        }
      }
      event "Icons": Mouse Down? {
        # "When mouse click on icons array - Do \"Action for specific icon\""
        n163 = event-data() -> ("CtlRef"=w507:refnum<vi>, "Coords"=w506:T21, "Button"=w499:u16)  [unwired: 1 in, 5 out]
        n164 = control-ref of="Icons Values"() -> (w498:refnum<vi>)
        n165 = call "GetArrayIndexFromCoordinate.vi"("error in (no error)"=w491, "Coords in"=w506, "Array in"=w507) -> ("error out"=w490:errorcluster, "in element? (1D arrays only)"=w494:bool, "Element Indexes"=w493:cluster{"Horizontal":u32, "Vertical":u32}, "Array out"=w505:refnum<vi>)  [unwired: 3 in, 2 out]
        n166 = property on="Property Node" class="Pnl"(reference=w495, error in=w490, "DeferPanUpdts"=FALSE ("Defer Panel Updates")) -> (error out=w497:errorcluster)  [unwired: 1 out]
        n167 = Unbundle By Name(w493) -> ("Horizontal"=w492:u32)
        n168 = control-ref of="IconNames"() -> (w501:refnum<vi>)
        n169 = case shown="True" w494 {
          tunnel: [w514 w538] -> w509
          tunnel: [w514 w537] -> w508
          tunnel: w505 -> [_ w523]
          tunnel: w492 -> [_ w522]
          tunnel: w497 -> [w513 w533]
          tunnel: [w513 w526] -> w504
          tunnel: w502 -> [w512 w532]
          tunnel: [w512 w531] -> w503
          tunnel: w501 -> [_ w518]
          tunnel: [w511 TRUE ("Discard?")] -> w500
          tunnel: w499 -> [w510 _]
          tunnel: w498 -> [_ w524]
          frame False {
            w514 = "" ("Empty String Constant")
            # "not in element"
            n170 = case "Mouse button" shown="1" w510 {
              tunnel: [TRUE ("Discard?") TRUE ("Discard?") FALSE ("Discard?")] -> w511
              frame 0 {
              }
              frame Default {
              }
              frame 1 {
              }
            }
          }
          frame True {
            # "in element"
            n171 = property on="Property Node" class="Arr (strict)"(reference=w518, error in=w533) -> (error out=w529:errorcluster, "Value"=w536:string[])  [unwired: 1 out]
            n172 = call "SwitchIconByNumber.vi"("Index"=w522, "error in (no error)"=w529, "Icon Array Ref"=w523, "Switch Values ref"=w524) -> ("error out"=w528:errorcluster, "Val out"=w519:bool, "Icon Array ref out"=w520:refnum<vi>, "Switch Values ref out"=w521:refnum<vi>)  [unwired: 4 in]
            n173 = Index Array(array=w536, index=w522) -> (element=w535:string)
            n174 = case "Action for specific icon" shown="\"zoom-to-actual-size\"" w535 {
              selector: w535 -> [w565 w580 w594 w603]
              tunnel: [w565 w580 w594 w603] -> w534
              tunnel: w528 -> [w562 w572 w587 w607]
              tunnel: [w562 w574 w592 w606] -> w527
              tunnel: w532 -> [w564 w566 w593 w605]
              tunnel: [w564 w575 w591 w604] -> w531
              tunnel: [w563 w579 w590 w602] -> w525
              tunnel: w519 -> [_ _ w585 w601]
              frame "Latch button name", Default {
                w563 = FALSE  # Switch(T)/Latch(F)
                (unwired) TRUE
                # "Duplicate this case for \"latch\" icon action"
                n175 = Wait (ms)(milliseconds to wait=u32 100) -> ()  [unwired: 1 out]
              }
              frame "zoom-to-actual-size" {
                w579 = FALSE  # Switch(T)/Latch(F)
                # "Note: Only ScaleFits visible objects!"
                # "Autoscale all graphs and resize objects in graph's pane (latch)"
                n176 = control-ref of="Intensity Graph"() -> (w568:refnum<vi>)
                n177 = control-ref of="Intensity Graph 2"() -> (w567:refnum<vi>)
                n178 = control-ref of="XY Graph"() -> (w570:refnum<vi>)
                n179 = control-ref of="XY Graph 2"() -> (w578:refnum<vi>)
                n180 = control-ref of="XY Graph 3"() -> (w577:refnum<vi>)
                n181 = Build Array(w570, w578, w577, w568, w567) -> (w576:refnum<vi>[])
                n182 = for {
                  tunnel: w576 -> [w584] mode=indexing
                  shift-right: [w581] -> w569
                  shift-left: w572 -> [w582]
                  w583 = u8 1 ("X Scale.Scale Fit")
                  n183 = property on="Property Node" class="GrphChrt"(reference=w584, error in=w582, "XScale.ScaleFit"=w583, "YScale.ScaleFit"=w583) -> (error out=w581:errorcluster)  [unwired: 1 out]
                }
                n184 = property on="Property Node" class="IntGraph (strict)"(reference=w567, error in=w569) -> (error out=w571:errorcluster, "OwningPane"=w573:refnum<vi>)  [unwired: 1 out]
                n185 = call-dynamic "ResizeObjectsinPane.vi"("error in (no error)"=w571, "PaneRef"=w573, "PentaPanesGUI in"=w566) -> ("error out"=w574:errorcluster, "PentaPanesGUI out"=w575:refnum<class "PentaPanes.lvclass">)  [unwired: 7 in]
              }
              frame "log" {
                w588 = T19 4 items=["Top", "Left", "Center", "Right", "Bottom"] ("Pane Position")
                w590 = TRUE  # Switch(T)/Latch(F)
                # "open/close bottom (log) pane (switch)"
                n186 = case "Switch new Value" shown="True" w585 {
                  tunnel: [0 ("t") w599] -> w589
                  tunnel: w587 -> [w595 w598]
                  tunnel: [w595 w597] -> w586
                  frame False {
                    # "Close Bottom Pane"
                  }
                  frame True {
                    # "Show Bottom Pane"
                    n187 = control-ref of="Bottom Pane Size"() -> (w600:refnum<vi>)
                    n188 = property on="Property Node" class="DigNum (strict)"(reference=w600, error in=w598) -> (error out=w597:errorcluster, "Value"=w599:i32)  [unwired: 1 out]
                  }
                }
                n189 = call "SetPaneSize.vi"("error in (no error)"=w586, "Pane Size"=w589, "Pane Position"=w588, "PentaPanesGUI in"=w593) -> ("error out"=w592:errorcluster, "PentaPanesGUI out"=w591:refnum<class "PentaPanes.lvclass">)  [unwired: 6 in]
              }
              frame "Switch button name" {
                w602 = TRUE  # Switch(T)/Latch(F)
                # "Duplicate this case for new \"switch\" icon actions"
                n190 = case "Switch new Value" shown="True" w601 {
                  tunnel: w607 -> [w609 w611]
                  tunnel: [w609 w611] -> w606
                  tunnel: w605 -> [w608 w610]
                  tunnel: [w608 w610] -> w604
                  tunnel: w603 -> [_ _]
                  frame False {
                    # "New Button Value - False"
                  }
                  frame True {
                    # "New Button Value - True"
                  }
                }
              }
            }
            n191 = flat-sequence "Log Line Builder" {
              tunnel: ["" ("Empty String Constant")] -> w538
              tunnel: w522 -> [w557]
              tunnel: [w558] -> w537
              tunnel: w534 -> [w554]
              tunnel: w525 -> [w553]
              tunnel: w519 -> [w552]
              frame #0 {
                n192 = Select(t="On" ("string"), s=w552, f="Off" ("string")) -> (s? t:f=w548:string)
                n193 = Number To Decimal String(number=w557) -> (decimal integer string=w556:string)  [unwired: 1 in]
                n194 = Concatenate Strings(" switched " ("string"), w548) -> (w547:string)
                n195 = Select(t=w547, s=w553, f=" pressed " ("string")) -> (s? t:f=w550:string)
                n196 = Concatenate Strings("Icon #" ("string"), w556, " " ("string"), w554, w550) -> (w558:string)
              }
            }
            n197 = case shown="False" w525 {
              tunnel: w527 -> [w543 w544]
              tunnel: [w542 w544] -> w526
              tunnel: w522 -> [w541 _]
              tunnel: w521 -> [w540 _]
              tunnel: w520 -> [w539 _]
              frame False {
                # "if Latch switch back off"
                n198 = call "SwitchIconByNumber.vi"("Index"=w541, "error in (no error)"=w543, "Icon Array Ref"=w539, "Switch Values ref"=w540) -> ("error out"=w542:errorcluster)  [unwired: 4 in, 3 out]
              }
              frame True {
              }
            }
          }
        }
        n199 = event-data ("Event Filter Node")("Discard?"=w500) -> ()  [unwired: 4 in, 1 out]
      }
      event "Options Tree": Value Change {
        # "When Tree Control changes value change to the tab page with the same name"
        n200 = event-data() -> ("NewVal"=w617:string[])  [unwired: 1 in, 5 out]
        n201 = Index Array(array=w617) -> (element=w616:string)  [unwired: 1 in]
        n202 = control-ref of="Options Tab"() -> (w623:refnum<vi>)
        n203 = property on="Property Node" class="TabCtl (strict)"(reference=w623, error in=w615) -> (reference out=w619:refnum<vi>, error out=w614:errorcluster, "Pages"=w622:refnum<vi>[])
        n204 = for {
          tunnel: w622 -> [w633] mode=indexing
          tunnel: w616 -> [w631]
          tunnel: [w630] -> w620 mode=indexing
          shift-right: [w628] -> w613
          shift-left: w614 -> [w629]
          n205 = property on="Property Node" class="Page"(reference=w633, error in=w629) -> (error out=w628:errorcluster, "PageLabel"=w632:string)  [unwired: 1 out]
          n206 = Equal?(x=w631, y=w632) -> (x = y?=w630:bool)
        }
        n207 = Search 1D Array(1D array=w620, element=TRUE) -> (index of element=w618:i32)  [unwired: 1 in]
        n208 = property on="Property Node" class="TabCtl (strict)"(reference=w619, error in=w613, "Value"=w618) -> (error out=w612:errorcluster)  [unwired: 1 out]
        n209 = flat-sequence "Log Line Builder" {
          tunnel: ["Set Settings Tab to: " ("String")] -> w627
          tunnel: [w634] -> w626
          tunnel: w612 -> [w635]
          tunnel: [w635] -> w625
          tunnel: w616 -> [w634]
          frame #0 {
          }
        }
      }
      event Panel Close? {
        w641 = TRUE  # Discard? T - Don't close panel.
        # "Shutdown and quit"
        n210 = event-data() -> ()  [unwired: 1 in, 4 out]
        n211 = event-data ("Event Filter Node")("Discard?"=w641) -> ()  [unwired: 1 in, 1 out]
      }
      event "Intensity Graph 2", "Intensity Graph": Scale Range Change {
        # "When intensity graph range changes resize pane objects (in order to keep correct aspect ratio)"
        n212 = event-data() -> ("CtlRef"=w649:refnum<vi>, "ScaleRef"=w646:refnum<vi>, "NewRange"=w645:T22)  [unwired: 1 in, 5 out]
        n213 = property on="Property Node" class="IntGraph (strict)"(reference=w649, error in=w644) -> (reference out=w647:refnum<vi>, error out=w643:errorcluster, "OwningPane"=w648:refnum<vi>)
        n214 = call-dynamic "ResizeObjectsinPane.vi"("error in (no error)"=w643, "PaneRef"=w648, "PentaPanesGUI in"=w652) -> ("error out"=w650:errorcluster, "PentaPanesGUI out"=w651:refnum<class "PentaPanes.lvclass">)  [unwired: 7 in]
        n215 = flat-sequence "Log Line Builder" {
          tunnel: [w668] -> w655
          tunnel: ["" ("Empty String Constant")] -> w654
          tunnel: w650 -> [w658]
          tunnel: [w669] -> w653
          tunnel: w647 -> [w666]
          tunnel: w646 -> [w665]
          tunnel: w645 -> [w664]
          frame #0 {
            n216 = property on="Property Node" class="IntGraph (strict)"(reference=w666, error in=w658) -> (error out=w657:errorcluster, "Label.Text"=w663:string)  [unwired: 1 out]
            n217 = property on="Property Node" class="GrphScl"(reference=w665, error in=w657) -> (error out=w656:errorcluster, "NameLbl.Text"=w662:string)  [unwired: 1 out]
            n218 = Unbundle By Name(w664) -> ("Minimum"=w660:dbl, "Maximum"=w659:dbl)
            n219 = Format Into String(format string="Intensity graph \"%s\" axis %s range set: %f %f" ("decimal integer string"), error in=w656, w663, w662, w660, w659) -> (resulting string=w668:string, error out=w669:errorcluster)  [unwired: 1 in]
          }
        }
      }
      event Panel Resize {
        # "Front Panel resized"
        n220 = event-data() -> ()  [unwired: 1 in, 8 out]
        n221 = flat-sequence "Log Line Builder" {
          tunnel: [w682] -> w673
          tunnel: w672 -> [w681]
          tunnel: [w680] -> w671
          tunnel: ["FrontPanel resized " ("String")] -> w670
          frame #0 {
            n222 = control-ref of="FP Bounds"() -> (w678:refnum<vi>)
            n223 = call "ClusterToDescriptiveString.vi"("error in"=w681, "Cluster In"=w678) -> ("error out"=w680:errorcluster, "String"=w682:string)  [unwired: 8 in]
          }
        }
        n224 = call "GetFPInfo.vi"("error in (no error)"=w675, "PentaPanesGUI in"=w677) -> ("error out"=w672:errorcluster, "Bounds"=→"FP Bounds":T13, "PentaPanesGUI out"=w676:refnum<class "PentaPanes.lvclass">)  [unwired: 6 in, 1 out]
      }
      event "Developed By\nLEAP CODE\nLinking hardware \nwith software\n\nYoni Cohen": Mouse Down {
        # "Opens icons8 website in default browser when clicking on link"
        n225 = event-data() -> ("Button"=w683:u16)  [unwired: 1 in, 7 out]
        n226 = case shown="1" w683 {
          tunnel: [w689 w694] -> w687
          tunnel: [w690 "Open Linkedin page: " ("String")] -> w686
          tunnel: w685 -> [w689 w692]
          tunnel: [w690 w691] -> w684
          frame 0, Default {
            w690 = "" ("String")
          }
          frame 1 {
            w691 = "https://www.linkedin.com/in/yoni-cohen-a03421110/"
            n227 = call-poly <vilib>:"Open URL in Default Browser.vi"("error in (no error)"=w692, "URL"=w691) -> ("error out"=w694:errorcluster)  [unwired: 4 in, 1 out]
          }
        }
      }
      event "Icon set by": Mouse Down {
        # "Opens icons8 website in default browser when clicking on link"
        n228 = event-data() -> ("CtlRef"=w700:refnum<vi>)  [unwired: 1 in, 7 out]
        n229 = property on="Property Node" class="Str"(reference=w700, error in=w696) -> (error out=w695:errorcluster, "Text.Text"=w697:string)  [unwired: 1 out]
        n230 = call-poly <vilib>:"Open URL in Default Browser.vi"("error in (no error)"=w695, "URL"=w697) -> ("error out"=w699:errorcluster)  [unwired: 4 in, 1 out]
      }
    }
    n231 = control-ref of="Listbox"() -> (w186:refnum<vi>)
    n232 = call "AddTextLineToListBox.vi"("error in (no error)"=w178, "String2"=w179, "String"=w187, "ListBox in"=w186) -> ("error out"=w177:errorcluster)  [unwired: 7 in]
    "Eventloop Error" <- w177
    n233 = call <vilib>:"Simple Error Handler.vi"("error in (no error)"=w177) -> ()  [unwired: 4 in, 5 out]
  }
  n234 = call "ShutDown5Panes.vi"("error in (no error)"=w30, "PentaPanesGUI in"=w28) -> ("error out"=w27:errorcluster)  [unwired: 9 in]
  n235 = call <vilib>:"Simple Error Handler.vi"("error in (no error)"=w27) -> ()  [unwired: 4 in, 5 out]
  "Init Error" <- w14
